vi "TCPPacket Read Header.vi"(8 "error in (no error)":errorcluster, 10 "Data":u8[](array[numeric]), 11 "TCPPacket in":refnum<class "TCPPacket.lvclass">) -> (0 "error out":errorcluster, 3 "TCPPacket out":refnum<class "TCPPacket.lvclass">)   [LabVIEW 2019, in "TCPPacket.lvclass"]
uses:
  TCPPacket.lvclass
  <vilib>/addons/Tools/Unicode/UTF8 Tools.lvlib
  <vilib>/addons/_JKI.lib/Serialization/JSON/JKI JSON Serialization.lvlib
  TCPHeader STYP.ctl
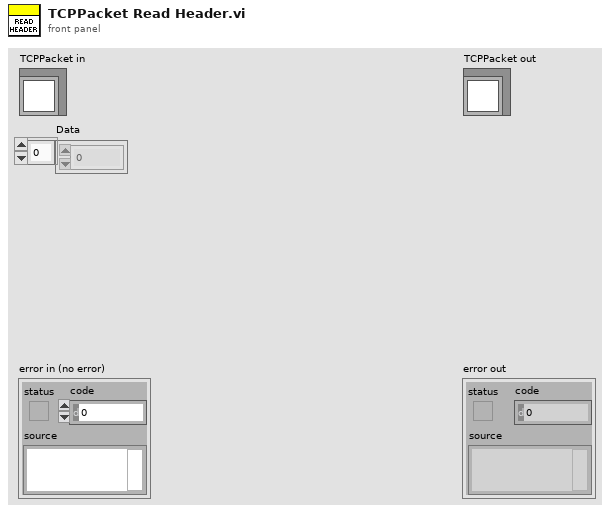
[diagram p1: front panel]
types:
  T1 = typedef "TCPPacket.lvclass/TCPHeader STYP.ctl" = cluster{"byteorder":string, "content-length":u32, "content-type":string, "content-encoding":string}
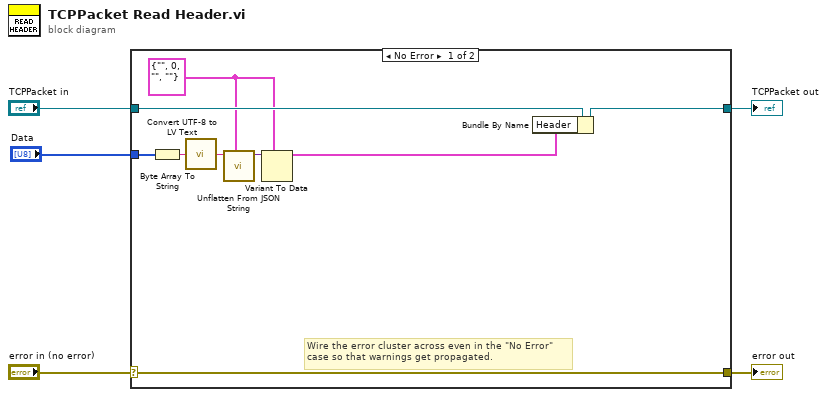
[diagram p0: block diagram]
diagram:
  n1 = case shown="No Error" "error in (no error)" {
    selector: "error in (no error)" -> [w13 w16]
    tunnel: [w13 w16] -> w4
    tunnel: [w7 w15] -> w2
    tunnel: "TCPPacket in" -> [w14 w15]
    tunnel: "Data" -> [w12 _]
    frame No Error {
      w8 = T1 {"byteorder"="", "content-length"=0, "content-type"="", "content-encoding"=""} ("Header")
      # "Wire the error cluster across even in the \"No Error\"\ncase so that warnings get propagated."
      n2 = Byte Array To String(unsigned byte array=w12) -> (string=w11:string)
      n3 = call <vilib>:"Convert UTF-8 to LV Text.vi"("UTF-8 Text"=w11) -> ("LV Text"=w10:string)  [unwired: 13 in, 1 out]
      n4 = call <vilib>:"Unflatten From JSON String.vi"("Type and Defaults"=w8, "JSON String"=w10) -> ("Variant"=w9:variant)  [unwired: 8 in, 1 out]
      n5 = Variant To Data(type=w8, Variant=w9) -> (data=w6:T1)  [unwired: 1 in, 1 out]
      n6 = Bundle By Name(cluster=w14, "Header"=w6) -> (w7:refnum<class "TCPPacket.lvclass">)
    }
    frame Error {
    }
  }
  "error out" <- w4
  "TCPPacket out" <- w2
